vi "Logging Equals.vi"   [LabVIEW 2012, in "femtoRoboLib.lvlib"]
uses:
  femtoRoboLib.lvlib
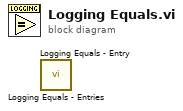
[diagram p0: block diagram]
diagram:
  n1 = call "Logging Equals - Entries.vi"() -> ()  [unwired: 6 in, 1 out]
  n2 = call "Logging Equals - Entry.vi"() -> ()  [unwired: 6 in, 1 out]
